vi "PlotSPIKEData.vi"(9 "offset":i32, 10 "Spike Data":string, 11 "wait (sec)":dbl=0.005) -> (3 "Closed Loop Step Response":cluster{"time":dbl[], dbl[]}[](graph))   [LabVIEW 2024]
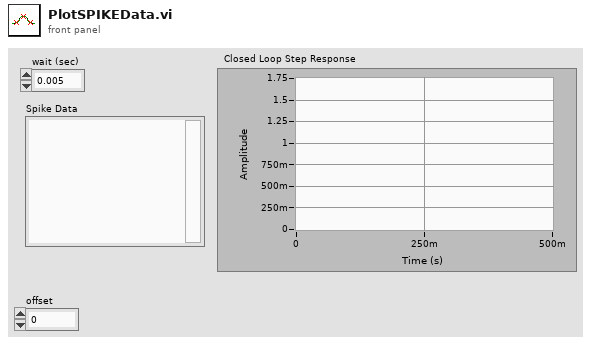
[diagram p1: front panel]
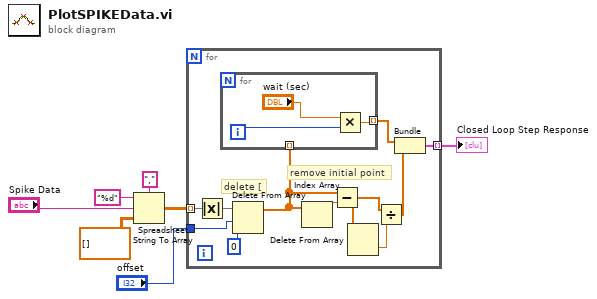
[diagram p0: block diagram]
diagram:
  n1 = Spreadsheet String To Array(delimiter (Tab)=",", format string="%d", spreadsheet string="Spike Data", array type (2D Dbl)=dbl[][] []) -> (array=w5:dbl[][])
  n2 = for {
    tunnel: w5 -> [w16] mode=indexing
    tunnel: [w13] -> w6 mode=indexing
    tunnel: "offset" -> [w8]
    # "remove initial point"
    # "delete ["
    n3 = Absolute Value(x=w16) -> (abs(x)=w12:dbl[])
    n4 = Delete From Array(array=w12, length=w8, index=0) -> (array with subset deleted=w14:dbl[])  [unwired: 1 out]
    n5 = for {
      tunnel: [w21] -> w15 mode=indexing
      tunnel: w14 -> [_] mode=indexing
      i -> [w20]
      n6 = Multiply(x="wait (sec)", y=w20) -> (x*y=w21:dbl)
    }
    n7 = Index Array(array=w14) -> (element=w18:dbl)  [unwired: 1 in]
    n8 = Subtract(x=w14, y=w18) -> (x-y=w10:dbl[])
    n9 = Delete From Array(array=w10) -> (deleted portion=w9:dbl)  [unwired: 2 in, 1 out]
    n10 = Divide(x=w10, y=w9) -> (x/y=w11:dbl[])
    n11 = Bundle(w15, w11) -> (w13:cluster{dbl[], dbl[]})  [unwired: 1 in]
  }
  "Closed Loop Step Response" <- w6
